vi "Get Header Data Start Index.vi"() -> (1 "Start Index[3]":u32[](array[numeric]))   [LabVIEW 8.6, in "Keyence LJ-V7000.lvlib"]
uses:
  Keyence LJ-V7000.lvlib
panel:
  # "Encoder Cnt"
  # "Encoder Z-in"
  # "Trigger Cnt"
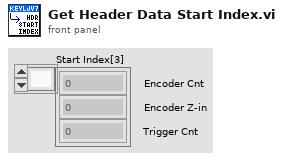
[diagram p1: front panel]
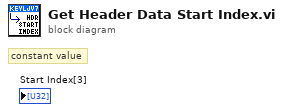
[diagram p0: block diagram]
diagram:
  # "constant value"
